vi "bead-center-x-correlation-simple-sum-v2(完成).vi"(0 "Image Pixels (U8)":u8[][](array[numeric]), 1 "Scan Window Size":i32=20, 2 "Lines  amount":i32=20, 3 "error in (no error) 2":errorcluster caption="错误输入（无错误）", 4 "half length fitting":i32=1) -> (5 "center coordinate x":dbl, 6 "Fit@peak\nerror":bool, 7 "error out 2":errorcluster caption="错误输出")   [LabVIEW 2013]
uses:
  bead-center-x-correlation-simple-sum-v2.ctl
  <vilib>/gmath/NI_Gmath.lvlib
panel:
  in  "传递变量":T1={"Lines amount"=20, "Image Pixels (U8)"=[], "IP_row_采样起点"=0, "IP_column_number"=0, "sum of row"=[], "scan window"=[], "线性相关系数"=[], "执行结束？"=FALSE}
  out "XY Graphs":cluster{i32[], dbl[]}(graph)
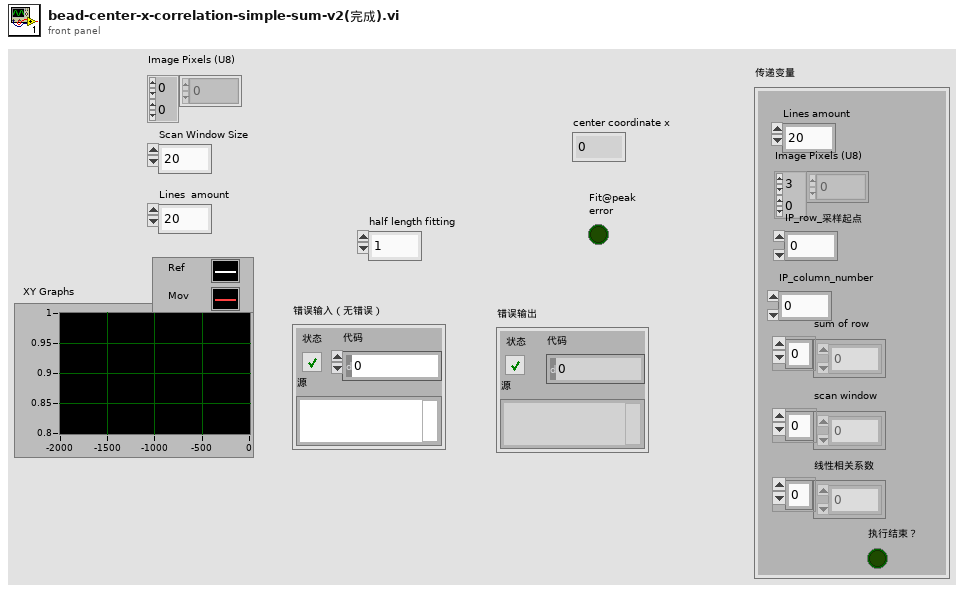
[diagram p1: front panel]
types:
  T1 = cluster{"Lines amount":i32, "Image Pixels (U8)":u8[][], "IP_row_采样起点":i32, "IP_column_number":i32, "sum of row":dbl[], "scan window":i32[], "线性相关系数":dbl[], "执行结束？":bool}
  T2 = typedef "bead-center-x-correlation-simple-sum-v2.ctl" = enum16{"初始化", "数组求和", "自相关", "算出X中心位置"}
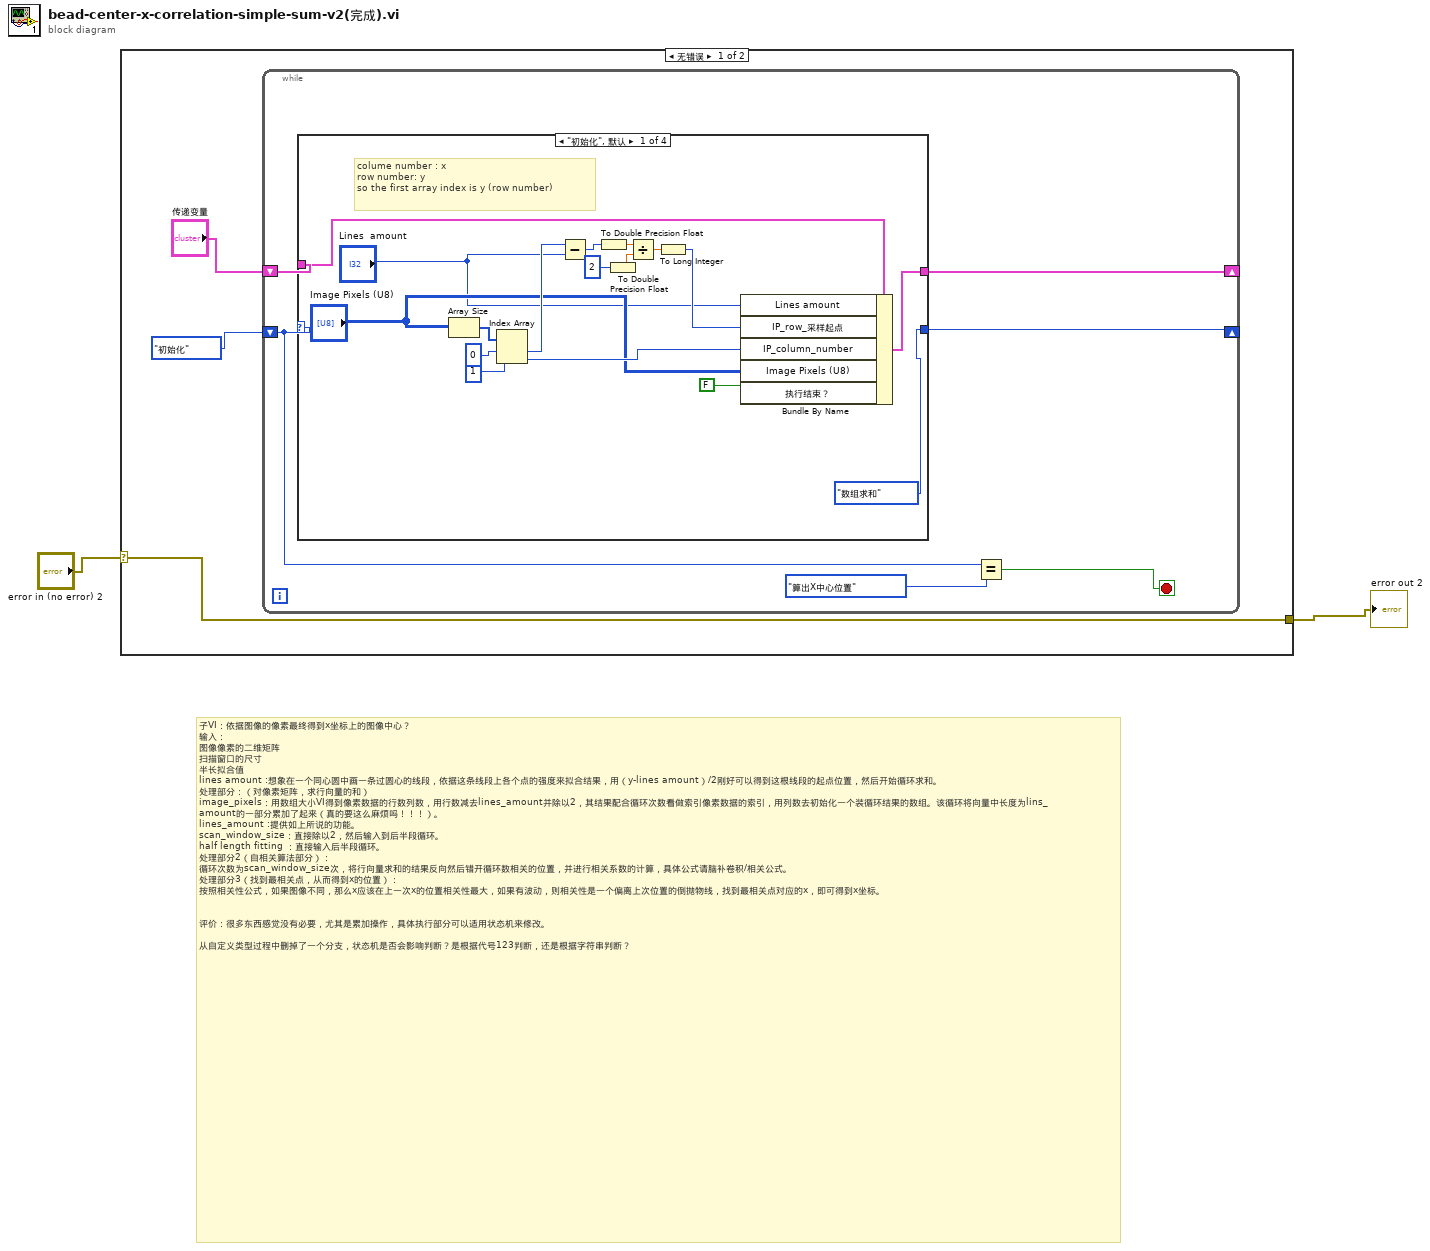
[diagram p0: block diagram]
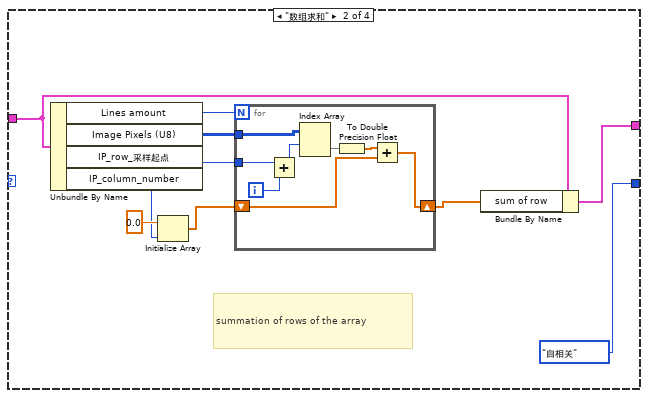
[diagram p2: hidden frame]
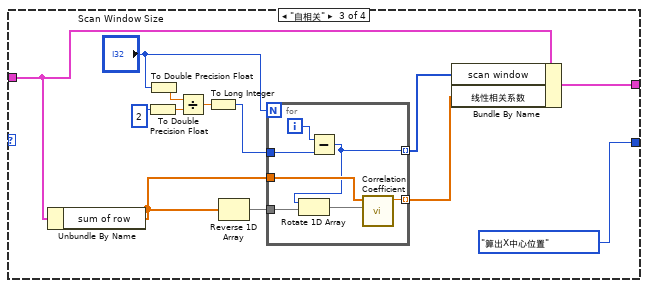
[diagram p3: hidden frame]
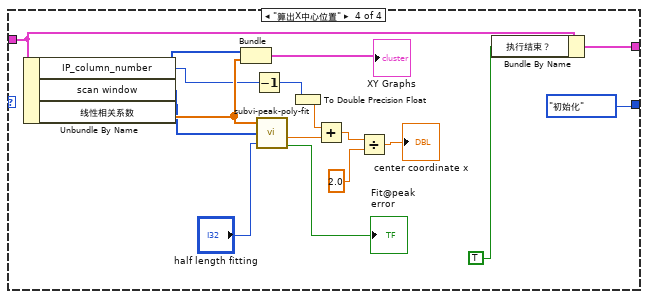
[diagram p4: hidden frame]
diagram:
  # "子VI：依据图像的像素最终得到x坐标上的图像中心？\n输入：\n图像像素的二维矩阵\n扫描窗口的尺寸\n半长拟合值\nlines amount :想象在一个同心圆中画一条过圆心的线段，依据这条线段上各个点的强度来拟合结果，用（y-lines amount）/2刚好可以得到这根线段的起点位置，然后开始循环求和。\n处理部分：（对像素矩阵，求行向量的和）\nimage_pixels：用数组大小VI得到像素数据的行数列数，用行数减去lines_amount并除以2，其结果配合循环次数看做索引像素数据的索引，用列数去初始化一个装循环结果的数组。该循环将向量中长度为lins_amount的一部分累加了起来（真的要这么麻烦吗！！！）。\nlines_amount :提供如上所说的功能。\nscan_window_size：直接除以2，然后输入到后半段循环。\nhalf length fitting ：直接输入后半段循环。\n处理部分2（自相关算法部分）：\n循环次数为scan_window_size次，将行向量求和的结果反向然后错开循环数相关的位置，并进行相关系数的计算，具体公式请脑补卷积/相关公式。\n处理部分3（找到最相关点，从而得到x的位置）：\n按照相关性公式，如果图像不同，那么x应该在上一次x的位置相关性最大，如果有波动，则相关性是一个偏离上次位置的倒抛物线，找到最相关点对应的x，即可得到x坐标。\n\n\n评价：很多东西感觉没有必要，尤其是累加操作，具体执行部分可以适用状态机来修改。\n\n从自定义类型过程中删掉了一个分支，状态机是否会影响判断？是根据代号123判断，还是根据字符串判断？"
  n1 = case shown="无错误" "error in (no error) 2" {
    selector: "error in (no error) 2" -> [w5 w83]
    tunnel: [w5 w83] -> w1
    frame No Error {
      n2 = while {
        shift-right: [w11] -> _
        shift-left: bead-center-x-correlation-simple-sum-v2."初始化" -> [w8]
        shift-right: [w9] -> _
        shift-left: "传递变量" -> [w10]
        stop <- w6 stop-if-true
        n3 = case shown="\"初始化\", 默认" w8 {
          tunnel: [bead-center-x-correlation-simple-sum-v2."数组求和" bead-center-x-correlation-simple-sum-v2."自相关" bead-center-x-correlation-simple-sum-v2."算出X中心位置" bead-center-x-correlation-simple-sum-v2."初始化"] -> w11
          tunnel: [w21 w29 w47 w67] -> w9
          tunnel: w10 -> [w17 w31 w50 w69]
          frame "初始化", Default {
            # "colume number : x\nrow number: y\nso the first array index is y (row number)"
            n4 = Array Size(array="Image Pixels (U8)") -> (size(s)=w23:i32[])
            n5 = Index Array(array=w23, index #1=0 ("index"), index #2=1 ("index")) -> (element #1=w20:i32, element #2=w15:i32)
            n6 = Subtract(x=w20, y="Lines  amount") -> (x-y=w28:i32)
            n7 = To Double Precision Float(number=w28) -> (double precision float=w19:dbl)
            n8 = To Double Precision Float(number=2 ("y")) -> (double precision float=w18:dbl)
            n9 = Divide(x=w19, y=w18) -> (x/y=w27:dbl)
            n10 = To Long Integer(number=w27) -> (32bit integer=w16:i32)
            n11 = Bundle By Name(cluster=w17, "Lines amount"="Lines  amount", "IP_row_采样起点"=w16, "IP_column_number"=w15, "Image Pixels (U8)"="Image Pixels (U8)", "执行结束？"=FALSE) -> (w21:T1)
          }
          frame "数组求和" {
            # "summation of rows of the array"
            n12 = Unbundle By Name(w31) -> ("Lines amount"=w35:i32, "Image Pixels (U8)"=w33:u8[][], "IP_row_采样起点"=w34:i32, "IP_column_number"=w30:i32)
            n13 = Initialize Array(0.0 ("element"), w30) -> (w38:dbl[])
            n14 = for {
              N: w35 -> [_]
              shift-right: [w45] -> w36
              shift-left: w38 -> [w46]
              tunnel: w34 -> [w42]
              tunnel: w33 -> [w41]
              i -> [w44]
              n15 = Add(x=w42, y=w44) -> (x+y=w39:i32)
              n16 = Index Array ("索引数组")(array=w41, index (row)=w39) -> (element=w40:u8[])  [unwired: 1 in]
              n17 = To Double Precision Float(number=w40) -> (double precision float=w43:dbl[])
              n18 = Add(x=w43, y=w46) -> (x+y=w45:dbl[])
            }
            n19 = Bundle By Name(cluster=w31, "sum of row"=w36) -> (w29:T1)
          }
          frame "自相关" {
            n20 = Unbundle By Name(w50) -> ("sum of row"=w53:dbl[])
            n21 = To Double Precision Float(number=2 ("y")) -> (double precision float=w52:dbl)
            n22 = To Double Precision Float(number="Scan Window Size") -> (double precision float=w51:dbl)
            n23 = Divide(x=w51, y=w52) -> (x/y=w55:dbl)
            n24 = To Long Integer(number=w55) -> (32bit integer=w56:i32)
            n25 = Reverse 1D Array(array=w53) -> (reversed array=w57:dbl[])
            n26 = for {
              N: "Scan Window Size" -> [_]
              tunnel: w57 -> [w66]
              tunnel: w53 -> [w65]
              tunnel: [w63] -> w48 mode=indexing
              tunnel: [w61] -> w49 mode=indexing
              tunnel: w56 -> [w60]
              i -> [w62]
              n27 = Subtract(x=w62, y=w60) -> (x-y=w61:i32)
              n28 = Rotate 1D Array(1:w66, 2:w61) -> (0:w64:dbl[])
              n29 = call <vilib>:"Correlation Coefficient.vi"("Y"=w64, "X"=w65) -> ("correlation coefficient r"=w63:dbl)  [unwired: 9 out]
            }
            n30 = Bundle By Name(cluster=w50, "scan window"=w49, "线性相关系数"=w48) -> (w47:T1)
          }
          frame "算出X中心位置" {
            n31 = Unbundle By Name(w69) -> ("IP_column_number"=w72:i32, "scan window"=w73:i32[], "线性相关系数"=w75:dbl[])
            n32 = Bundle("scan window"=w73, "线性相关系数"=w75) -> (→"XY Graphs":cluster{"scan window":i32[], "线性相关系数":dbl[]})  [unwired: 1 in]
            n33 = Decrement(x=w72) -> (x-1=w70:i32)
            n34 = call "subvi-peak-poly-fit .vi"("array_y"=w75, "array_x"=w73, "half length"="half length fitting") -> ("Max_x"=w76:dbl, "error"=→"Fit@peak\nerror":bool)  [unwired: 2 out]
            n35 = To Double Precision Float(number=w70) -> (double precision float=w71:dbl)
            n36 = Add(x=w71, y=w76) -> (x+y=w77:dbl)
            n37 = Divide(x=w77, y=2.0) -> (x/y=→"center coordinate x":dbl)
            n38 = Bundle By Name(cluster=w69, "执行结束？"=TRUE ("y")) -> (w67:T1)
          }
        }
        n39 = Equal?(x=w8, y=bead-center-x-correlation-simple-sum-v2."算出X中心位置") -> (x = y?=w6:bool)
      }
    }
    frame Error {
    }
  }
  "error out 2" <- w1
